vi "Configure Digital Channel.vi"(4 "Threshold Value (1.0 V)":dbl=1.0, 6 "Threshold (0: CMOS 5V)":i32(ring) items=["CMOS 5V", "CMOS 3.3V", "CMOS 2.5V", "ECL", "PECL", "TTL", "User Defined", "Differential"], 7 "Enable Channel (T: Enable)":bool=TRUE, 8 "error in (no error)":errorcluster, 9 "Size (1: Medium)":i32(ring)=1 items=["Small", "Medium", "Large"], 10 "Channel (20: DIG 0)":i32(ring)=20 items=["DIG 0"=20, "DIG 1"=21, "DIG 2"=22, "DIG 3"=23, "DIG 4"=24, "DIG 5"=25, "DIG 6"=26, "DIG 7"=27, "DIG 8"=28, "DIG 9"=29, "DIG 10"=30, "DIG 11"=31, "DIG 12"=32, "DIG 13"=33, "DIG 14"=34, "DIG 15"=35], 11 "VISA resource name":refnum<visa-resource-name>) -> (0 "error out":errorcluster, 3 "VISA resource name out":refnum<visa-resource-name>)   [LabVIEW 2020, in "Agilent 90000 Series.lvlib"]
doc: "Configures the common properties of the digital channels.\n\n<B>Note:</B>\nOnly valid for MSO models or DSO models with MSO license."
uses:
  Agilent 90000 Series.lvlib
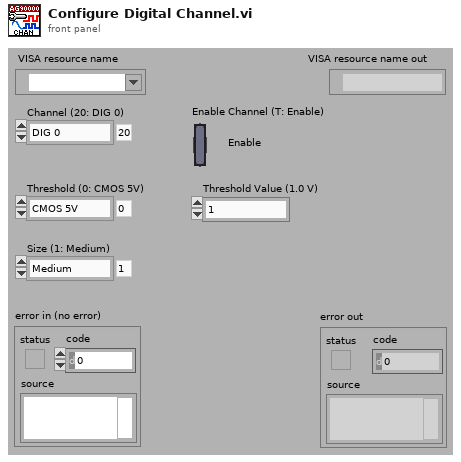
[diagram p1: front panel]
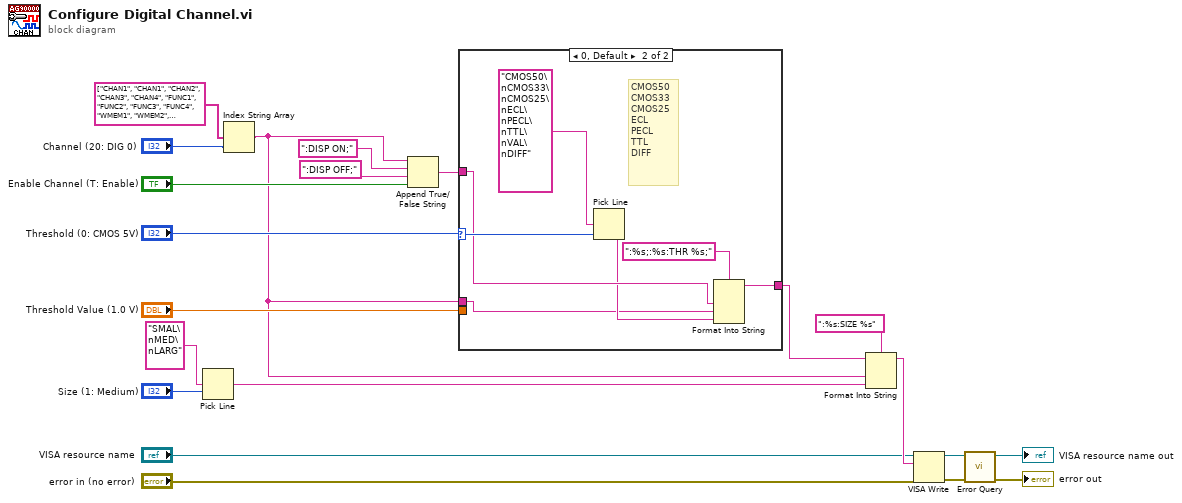
[diagram p0: block diagram]
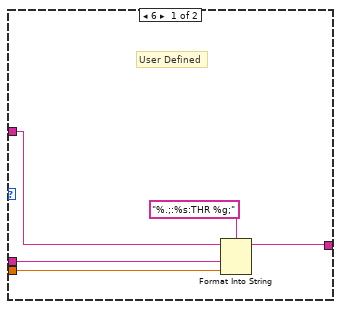
[diagram p2: hidden frame]
diagram:
  n1 = Pick Line(multi-line string="SMAL\nMED\nLARG", line index="Size (1: Medium)") -> (output string=w8:string)  [unwired: 1 out]
  n2 = Index String Array(1:"Channel (20: DIG 0)", 2:string[] ["CHAN1", "CHAN1", "CHAN2", "CHAN3", "CHAN4", "FUNC1", "FUNC2", "FUNC3", "FUNC4", "WMEM1", "WMEM2", "WMEM3", "WMEM4", "AUX", "LINE", "CLOC", "MTR", "MSP", "EQU", "NONE", "DIG0", "DIG1", "DIG2", "DIG3", "DIG4", "DIG5", "DIG6", "DIG7", "DIG8", "DIG9", "DIG10", "DIG11", "DIG12", "DIG13", "DIG14", "DIG15", "", "", "", "", "", "POD1", "POD2", "", "", "", "", "", "", "", "", "BUS1", "BUS2", "BUS3", "BUS4", "", "", "", "", "", "", "DIFF1", "DIFF2", "", "", "", "", "", "", "", "", "COMM3", "COMM4"]) -> (0:w1:string)  [unwired: 1 out]
  n3 = Append True/False String(1:"Enable Channel (T: Enable)", 2:":DISP OFF;" ("false string"), 3:":DISP ON;" ("true string"), 4:w1) -> (0:w13:string)
  n4 = case shown="0, Default" "Threshold (0: CMOS 5V)" {
    selector: "Threshold (0: CMOS 5V)" -> [_ w30]
    tunnel: "Threshold Value (1.0 V)" -> [w25 _]
    tunnel: w1 -> [w24 w27]
    tunnel: w13 -> [w22 w29]
    tunnel: [w23 w31] -> w4
    frame 6 {
      # "User Defined"
      n5 = Format Into String(format string="%.;:%s:THR %g;", initial string=w22, w24, w25) -> (resulting string=w23:string)  [unwired: 1 in, 1 out]
    }
    frame 0, Default {
      # "CMOS50\nCMOS33\nCMOS25\nECL\nPECL\nTTL\nDIFF"
      n6 = Pick Line(multi-line string="CMOS50\nCMOS33\nCMOS25\nECL\nPECL\nTTL\nVAL\nDIFF", line index=w30) -> (output string=w28:string)  [unwired: 1 out]
      n7 = Format Into String(format string=":%s;:%s:THR %s;", w29, w27, w28) -> (resulting string=w31:string)  [unwired: 2 in, 1 out]
    }
  }
  n8 = Format Into String(format string=":%s:SIZE %s", initial string=w4, w1, w8) -> (resulting string=w7:string)  [unwired: 1 in, 1 out]
  n9 = VISA Write(VISA resource name="VISA resource name", write buffer=w7, error in (no error)="error in (no error)") -> (VISA resource name out=w19:refnum<visa-resource-name>, error out=w18:errorcluster)  [unwired: 1 out]
  n10 = call "Error Query.vi"("error in (no error)"=w18, "VISA resource name"=w19) -> ("error out"=→"error out":errorcluster, "VISA resource name out"=→"VISA resource name out":refnum<visa-resource-name>)  [unwired: 8 out]
